vi "rx_config.vi"(0 "HW parameters In":T3={"Device IP Address"="192.168.11.6", "Active Antenna"="RX1", "Carrier Frequency (Hz)"=915000000.0, "Gain (dB)"=10.0, "Trigger Level"=0.01, "Bandwidth (Hz)"=40000000.0, "Reference Position (%)"=10.0, "Capture Time (s)"=0.0004, "Simulate"=FALSE} {"Capture Time (s)" format="%.2p"; "Bandwidth (Hz)" format="%.2p"; "Trigger Level" format="%#.3p"; "Gain (dB)" format="%.2f"; "Carrier Frequency (Hz)" format="%.2p"}, 5 "Modulation Parameters In":T2 {"RX Parameters"."RX Sample Rate" items=["4M"]}, 7 "Queues In":T1, 11 "error in (no error)":errorcluster) -> (1 "coerced bandwidth":dbl, 2 "coerced carrier frequency (Hz)":dbl=100000.0 format="%#_6p", 3 "coerced gain (dB)":dbl format="%#_6f", 4 "HW parameters Out":T3={"Device IP Address"="192.168.11.6", "Active Antenna"="RX1", "Carrier Frequency (Hz)"=915000000.0, "Gain (dB)"=10.0, "Trigger Level"=0.01, "Bandwidth (Hz)"=40000000.0, "Reference Position (%)"=10.0, "Capture Time (s)"=0.0004, "Simulate"=FALSE} {"Capture Time (s)" format="%.2p"; "Bandwidth (Hz)" format="%.2p"; "Trigger Level" format="%#.3p"; "Gain (dB)" format="%.2f"; "Carrier Frequency (Hz)" format="%.2p"}, 6 "Modulation Parameters Out":T2 {"RX Parameters"."RX Sample Rate" items=["4M"]}, 8 "Queues Out":T1, 10 "Simulate":bool, 15 "error out":errorcluster)   [LabVIEW 2012, in "gds_hw_config.lvlib"]
uses:
  EE 497/LABS/SDR/control_type_defs.llb/rx_hw params.ctl
  EE 497/LABS/SDR/control_type_defs.llb/Queues.ctl
  gds_hw_config.lvlib
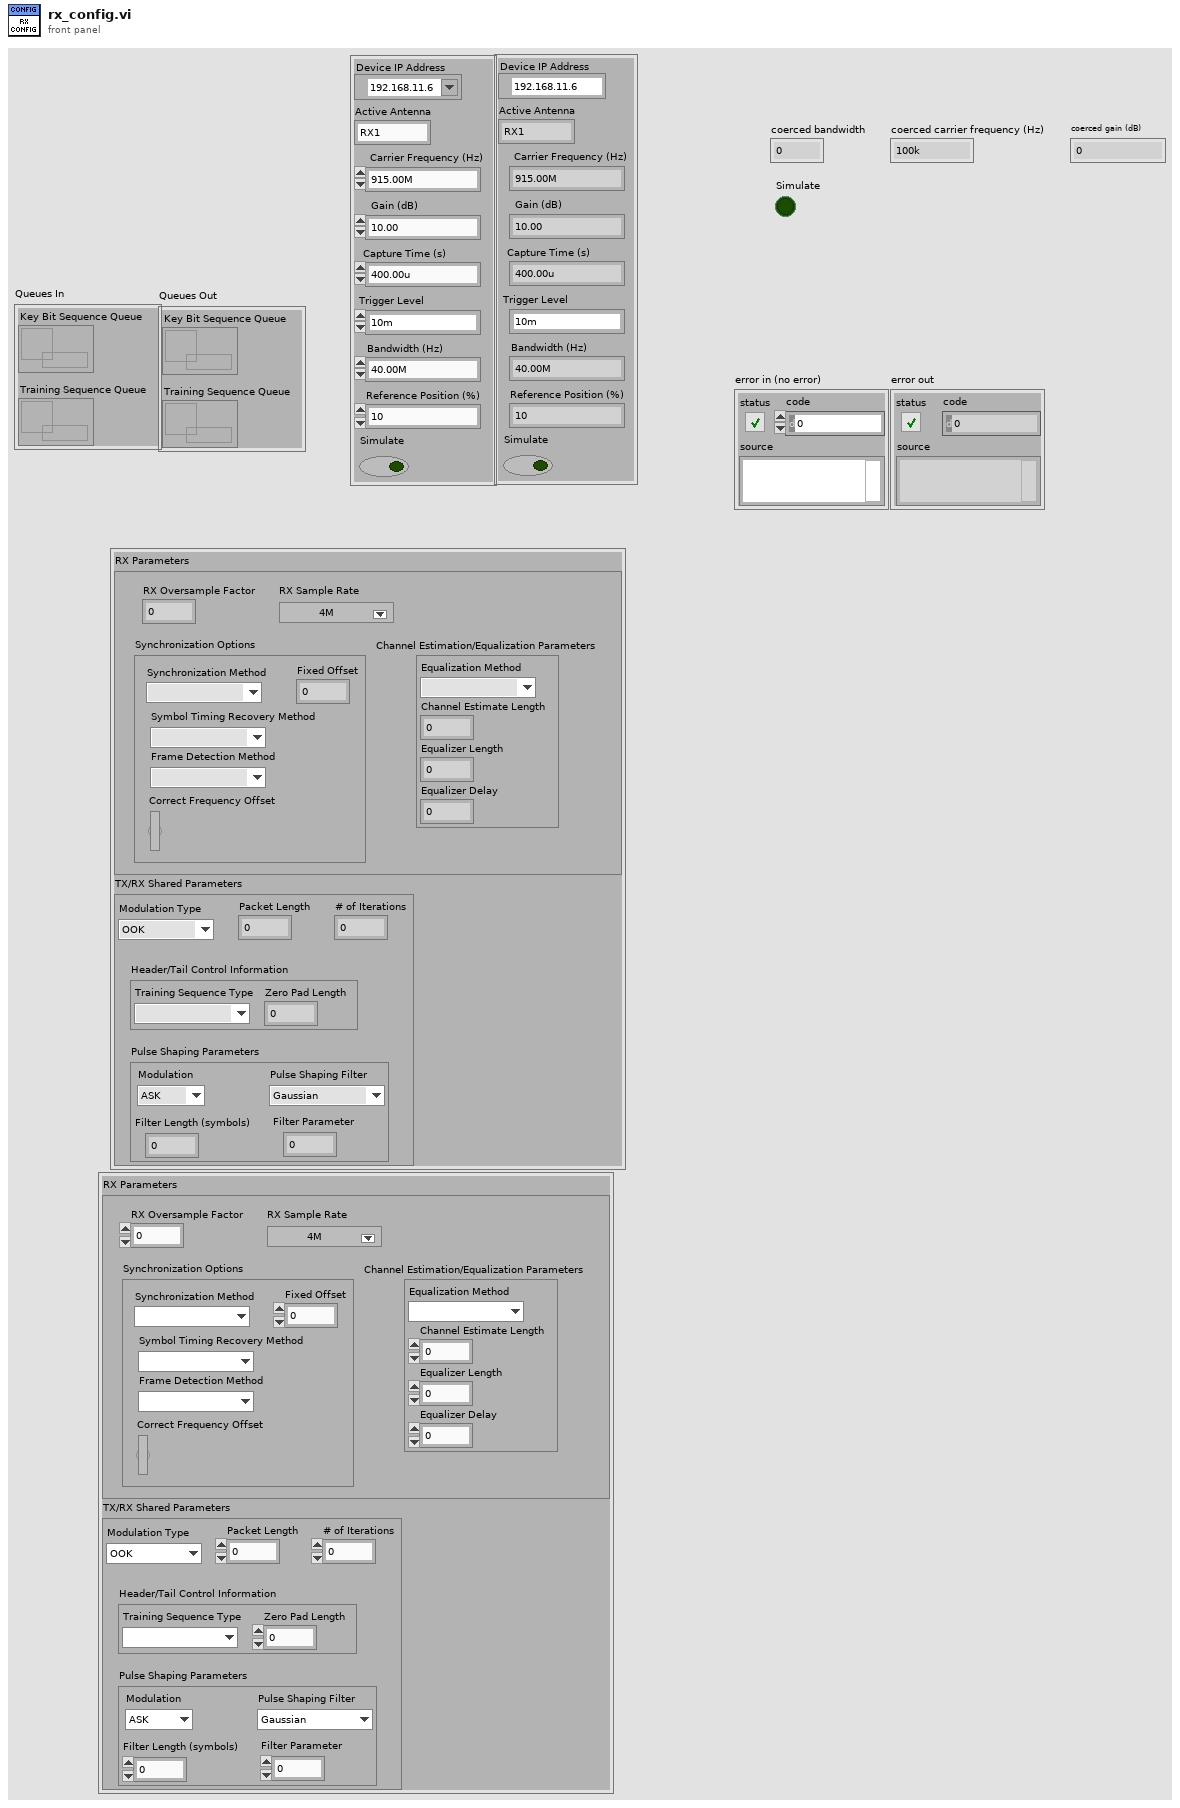
[diagram p1: front panel]
types:
  T1 = typedef "Queues.ctl" = cluster{"Key Bit Sequence Queue":refnum<queue>, "Training Sequence Queue":refnum<queue>}
  T2 = cluster{"RX Parameters":cluster{"RX Oversample Factor":dbl, "RX Sample Rate":dbl, "Synchronization Options":cluster{"Synchronization Method":enum16{""}, "Symbol Timing Recovery Method ":enum16{""}, "Fixed Offset":dbl, "Frame Detection Method":enum16{""}, "Correct Frequency Offset":bool}, "Channel Estimation/Equalization Parameters":cluster{"Equalization Method":enum16{""}, "Channel Estimate Length":dbl, "Equalizer Length":dbl, "Equalizer Delay":dbl}}, "TX/RX Shared Parameters":cluster{"Modulation Type":enum16{"OOK", "FSK"}, "Packet Length":dbl, "# of Iterations":dbl, "Pulse Shaping Parameters":cluster{"Modulation":enum16{"ASK", "FSK", "PSK", "QAM", "MSK", "PAM"}, "Pulse Shaping Filter":enum16{"Gaussian"}, "Filter Length (symbols)":dbl, "Filter Parameter":dbl}, "Header/Tail Control Information":cluster{"Training Sequence Type":enum16{""}, "Zero Pad Length":dbl}}}
  T3 = typedef "rx_hw params.ctl" = cluster{"Device IP Address":refnum<k15>, "Active Antenna":string, "Carrier Frequency (Hz)":dbl, "Gain (dB)":dbl, "Trigger Level":dbl, "Bandwidth (Hz)":dbl, "Reference Position (%)":dbl, "Capture Time (s)":dbl, "Simulate":bool}
  T4 = cluster{"RX Oversample Factor":dbl, "RX Sample Rate":dbl, "Synchronization Options":cluster{"Synchronization Method":enum16{""}, "Symbol Timing Recovery Method ":enum16{""}, "Fixed Offset":dbl, "Frame Detection Method":enum16{""}, "Correct Frequency Offset":bool}, "Channel Estimation/Equalization Parameters":cluster{"Equalization Method":enum16{""}, "Channel Estimate Length":dbl, "Equalizer Length":dbl, "Equalizer Delay":dbl}}
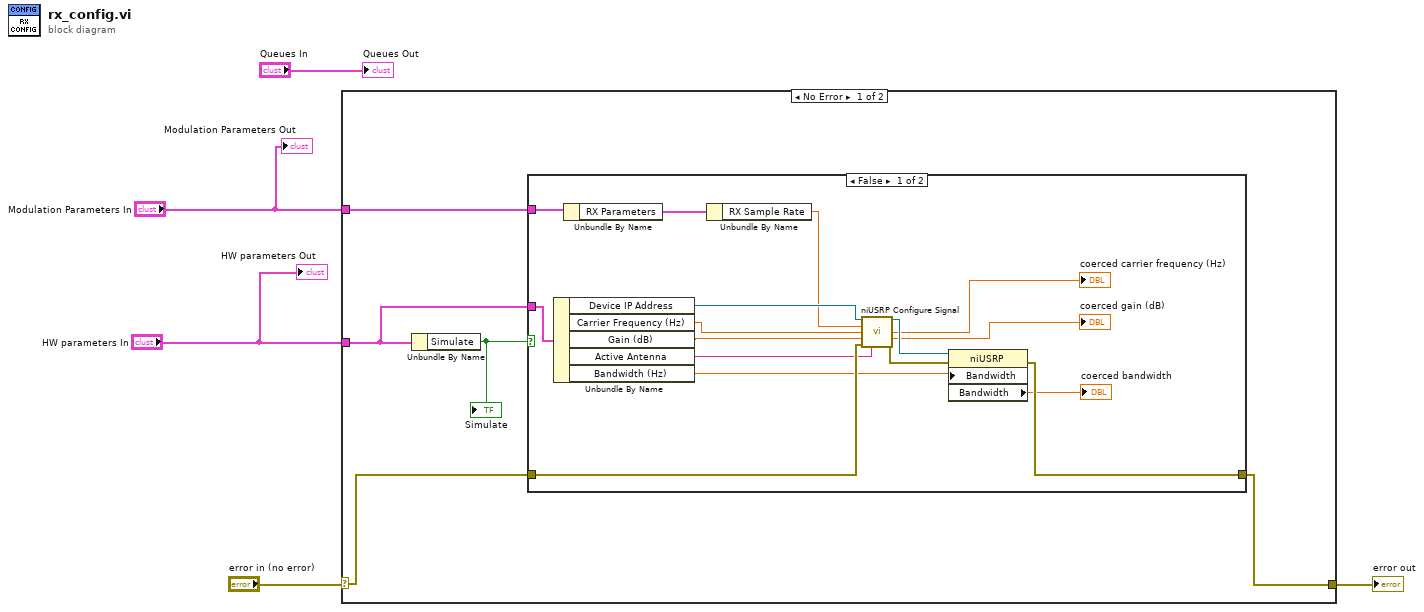
[diagram p0: block diagram]
diagram:
  n1 = case shown="No Error" "error in (no error)" {
    selector: "error in (no error)" -> [w10 w28]
    tunnel: [w9 w28] -> w4
    tunnel: "HW parameters In" -> [w8 _]
    tunnel: "Modulation Parameters In" -> [w7 _]
    frame No Error {
      n2 = Unbundle By Name(w8) -> ("Simulate"=w6:bool)
      "Simulate" <- w6
      n3 = case shown="False" w6 {
        tunnel: w10 -> [w21 w27]
        tunnel: [w14 w27] -> w9
        tunnel: w8 -> [w24 _]
        tunnel: w7 -> [w26 _]
        frame False {
          n4 = Unbundle By Name(w24) -> ("Device IP Address"=w23:refnum<k15>, "Carrier Frequency (Hz)"=w20:dbl, "Gain (dB)"=w19:dbl, "Active Antenna"=w18:string, "Bandwidth (Hz)"=w15:dbl)
          n5 = Unbundle By Name(w26) -> ("RX Parameters"=w25:T4)
          n6 = Unbundle By Name(w25) -> ("RX Sample Rate"=w22:dbl)
          n7 = call <instrlib>:"niUSRP Configure Signal.vi"("session handle"=w23, "IQ rate"=w22, "carrier frequency"=w20, "gain"=w19, "error in (no error)"=w21, "active antenna"=w18) -> ("session handle out"=w17:refnum<k15>, "coerced carrier frequency"=→"coerced carrier frequency (Hz)":dbl, "coerced gain"=→"coerced gain (dB)":dbl, "error out"=w16:errorcluster)  [unwired: 5 in, 1 out]
          n8 = property class="niUSRP"(reference=w17, error in=w16, "Bandwidth"=w15) -> (error out=w14:errorcluster, "Bandwidth"=→"coerced bandwidth":dbl)  [unwired: 1 out]
        }
        frame True {
        }
      }
    }
    frame Error {
    }
  }
  "error out" <- w4
  "HW parameters Out" <- "HW parameters In"
  "Modulation Parameters Out" <- "Modulation Parameters In"
  "Queues Out" <- "Queues In"
